vi "test1.vi"() -> ()   [LabVIEW 2017]
uses:
  <vilib>/userdefined/High Color/IMAQdx.ctl
  <vilib>/Platform/TimedLoop/XDataNode/timing_clust.ctl
  <vilib>/Platform/TimedLoop/XDataNode/nitl_modes.ctl
  <vilib>/Platform/TimedLoop/XDataNode/wakeup.ctl
  <vilib>/myRIO/Common/Instrument Driver Framework/myRIO v1.0/UART/vis/myRIO v1.0 Close UART.vi
  Global 1.vi
  Outputs.vi
  Inputs.vi
  <vilib>/myRIO/Common/Instrument Driver Framework/Utilities/vis/FPGA Ref Manager.vi
  <vilib>/myRIO/Common/Instrument Driver Framework/myRIO v1.0/myRIO v1.0 Reset FPGA.vi
  <vilib>/myRIO/Common/Instrument Driver Framework/myRIO v1.0/IRQ/vis/myRIO v1.0 IRQ Info FGV.vi
  <vilib>/myRIO/Common/Instrument Driver Framework/myRIO v1.0/IRQ/vis/myRIO v1.0 Timer IRQ Info FGV.vi
  <vilib>/myRIO/Common/Instrument Driver Framework/myRIO v1.0/IRQ/vis/myRIO v1.0 ISR Agent.vi
  <vilib>/platform/TimedLoop/XDataNode/XDataNode.xnode
  <vilib>/vision/driver/NI_Vision_Acquisition_Software.lvlib
  <vilib>/Platform/TimedLoop/XDataNode/XDNodeRunTimeDep.lvlib
  <vilib>/myRIO/Instrument Drivers/Utilities/Utilities.lvlib
panel:
  out "error out":errorcluster
  in  "Stop":bool
  out "Step":i16
  in  "Start":bool
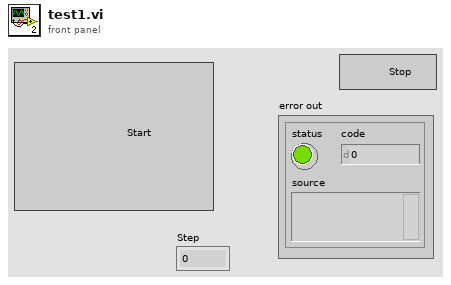
[diagram p1: front panel]
types:
  T1 = typedef "IMAQdx.ctl" = refnum<k21>
  T2 = typedef "XDNodeRunTimeDep.lvlib/timing_clust.ctl" = cluster{"Expected End [f-1]":u64, "Actual End [f-1]":u64, "Finished Late? [f-1]":bool, "Expected End [i-1]":u64, "Actual End [i-1]":u64, "Finished Late? [i-1]":bool, "Expected Start [i]":u64, "Actual Start [i]":u64, "Expected Start [f]":u64, "Actual Start [f]":u64, "Source Name":string, "Structure Name":string, "Period":i64, "Deadline":i64, "Offset":i64, "Start":i64, "Priority":i32, "Timeout":i32, "Mode":T3, "Wakeup Reason":T4, "Error":errorcluster, "Source Type":string, "Secondary Source Type":string, "Global End Time":u64, "Global Start Time":u64, "Frame Duration":u64, "Iteration Duration":u64, "Assigned CPU":i32, "I/O Scan Engine Mode":u32}
  T3 = typedef "XDNodeRunTimeDep.lvlib/nitl_modes.ctl" = enum32{"No Change", "Process missed periods, maintain original phase", "Discard missed periods, maintain original phase", "Process missed periods, ignore original phase", "Discard missed periods, ignore original phase"}
  T4 = typedef "XDNodeRunTimeDep.lvlib/wakeup.ctl" = enum32{"Normal", "Aborted", "Asynchronous wakeup", "Timing source error", "Timed loop error", "Timeout"}
  T5 = typedef "I2C.lvlib/I2C Reference.ctl" = cluster{"myRIO Reference":T6, "I2C Channels Enum":T10, "I2C Configuration":T11}
  T6 = typedef "myRIO Generic Hardware Reference.ctl" = cluster{"myRIO Model":T7, "myRIO Hardware Reference":T8}
  T7 = typedef "Hardware Version Enum.ctl" = enum16{"Unknown", "myRIO-1900", "myRIO-1950", "roboRIO", "NI ELVIS RIO CM"}
  T8 = typedef "myRIO v1.0 Reference.ctl" = cluster{"Generic FPGA Reference":T9, "Allow multiple opens":bool}
  T9 = typedef "Generic FPGA Reference.ctl" = refnum<k20>
  T10 = typedef "I2C Channels Enum.ctl" = enum16{"Not Connected", "A/I2C", "B/I2C", "I2C/I2C"}
  T11 = typedef "I2C.lvlib/I2C Configuration.ctl" = cluster{"I2C Transfer Rate":T12}
  T12 = typedef "I2C.lvlib/I2C Transfer Rate.ctl" = enum16{"Standard mode (100 kbps)", "Fast mode (400 kbps)"}
  T13 = typedef "IMAQ Image.ctl" = refnum<image>
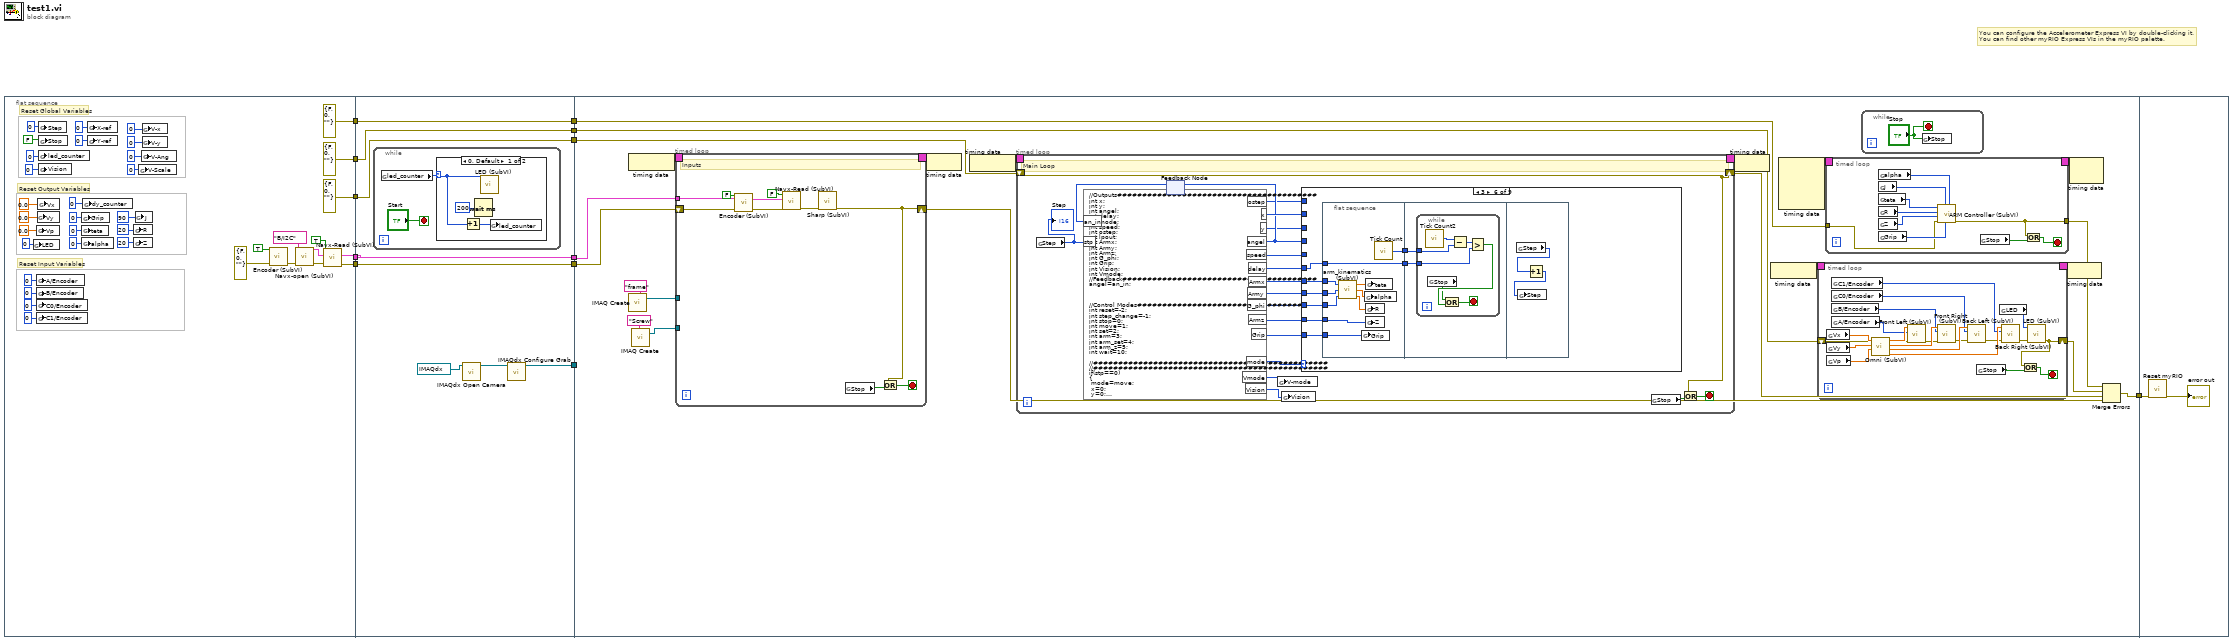
[diagram p0: block diagram]
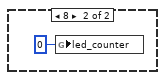
[diagram p2: hidden frame]
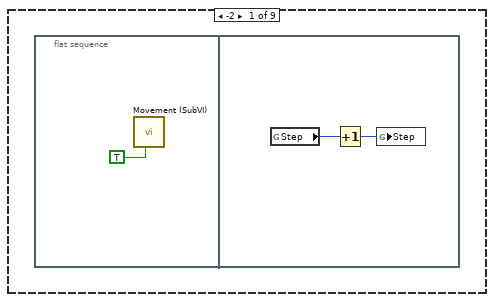
[diagram p3: hidden frame]
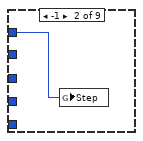
[diagram p4: hidden frame]
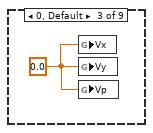
[diagram p5: hidden frame]
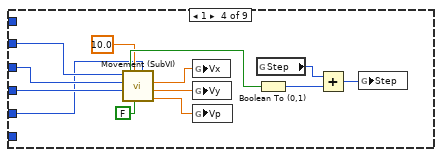
[diagram p6: hidden frame]
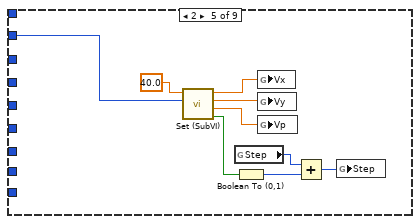
[diagram p7: hidden frame]
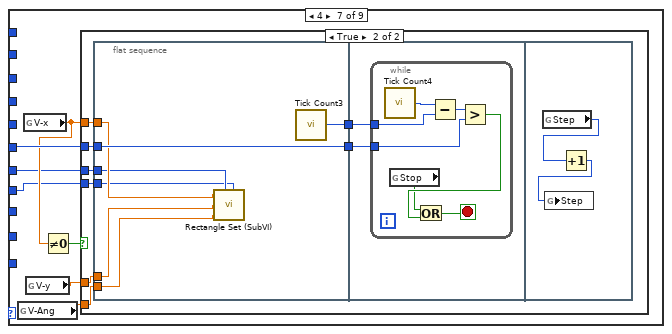
[diagram p8: hidden frame]
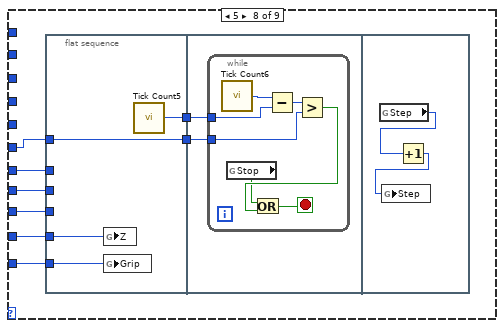
[diagram p10: hidden frame]
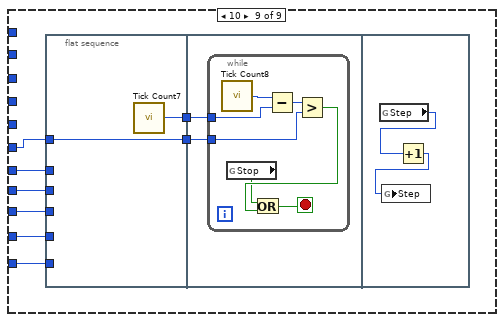
[diagram p11: hidden frame]
diagram:
  # "You can configure the Accelerometer Express VI by double-clicking it.\nYou can find other myRIO Express VIs in the myRIO palette."
  n1 = flat-sequence {
    tunnel: [w44] -> w12
    tunnel: [errorcluster {"status"=FALSE, "code"=0, "source"=""} ("error in (no error)")] -> w11
    tunnel: [errorcluster {"status"=FALSE, "code"=0, "source"=""} ("error in (no error)")] -> w10
    tunnel: [w42] -> w9
    tunnel: [errorcluster {"status"=FALSE, "code"=0, "source"=""} ("error in (no error)")] -> w8
    tunnel: w12 -> [w56]
    tunnel: [w56] -> w7
    tunnel: w11 -> [w55]
    tunnel: [w55] -> w6
    tunnel: w10 -> [w52]
    tunnel: w9 -> [w54]
    tunnel: [w54] -> w5
    tunnel: [w53] -> w4
    tunnel: w8 -> [w53]
    tunnel: [w52] -> w3
    tunnel: [w49] -> w2
    tunnel: w7 -> [w84]
    tunnel: w6 -> [w67]
    tunnel: w5 -> [w77]
    tunnel: w4 -> [w76]
    tunnel: [w75] -> w1
    tunnel: w3 -> [w68]
    tunnel: w2 -> [_]
    tunnel: w1 -> [w293]
    frame #0 {
      # "Reset Global Variables"
      # "Reset Input Variables"
      # "Reset Output Variables"
      # "Initialize"
      n2 = global write "Outputs.vi" "LED"(i8 0 ("LED")) -> ()
      n3 = global write "Outputs.vi" "Vp"(0.0 ("Vp")) -> ()
      n4 = global write "Inputs.vi" "A/Encoder"(0 ("A/Encoder")) -> ()
      n5 = global write "Inputs.vi" "B/Encoder"(0 ("B/Encoder")) -> ()
      n6 = global write "Inputs.vi" "C0/Encoder"(0 ("C0/Encoder")) -> ()
      n7 = global write "Inputs.vi" "C1/Encoder"(0 ("C1/Encoder")) -> ()
      n8 = global write "Outputs.vi" "Vy"(0.0 ("Vy")) -> ()
      n9 = global write "Outputs.vi" "Vx"(0.0 ("Vx")) -> ()
      n10 = global write "Global 1.vi" "Step"(i16 0 ("Step")) -> ()
      n11 = global write "Global 1.vi" "led_counter"(i8 0 ("Step")) -> ()
      n12 = global write "Global 1.vi" "Vision"(i8 0 ("Step")) -> ()
      n13 = global write "Global 1.vi" "Stop"(FALSE ("Stop")) -> ()
      n14 = global write "Outputs.vi" "Grip"(i16 0 ("Grip")) -> ()
      n15 = global write "Outputs.vi" "teta"(i16 0 ("teta")) -> ()
      n16 = global write "Outputs.vi" "alpha"(i16 0 ("alpha")) -> ()
      n17 = global write "Outputs.vi" "dy_counter"(i8 0 ("LED")) -> ()
      n18 = global write "Global 1.vi" "X-ref"(i64 0 ("X-ref")) -> ()
      n19 = global write "Global 1.vi" "Y-ref"(i64 0 ("Y-ref")) -> ()
      n20 = global write "Outputs.vi" "R"(i16 20 ("R")) -> ()
      n21 = global write "Outputs.vi" "Z"(i16 20 ("Z")) -> ()
      n22 = global write "Outputs.vi" "J"(i16 90 ("J")) -> ()
      n23 = global write "Global 1.vi" "V-Scale"(i64 0 ("Y-ref")) -> ()
      n24 = global write "Global 1.vi" "V-Ang"(i64 0 ("X-ref")) -> ()
      n25 = global write "Global 1.vi" "V-x"(i64 0 ("X-ref")) -> ()
      n26 = global write "Global 1.vi" "V-y"(i64 0 ("Y-ref")) -> ()
      n27 = call "Encoder (SubVI).vi"("error in (no error)"=errorcluster {"status"=FALSE, "code"=0, "source"=""}, "Reset?"=TRUE ("Reset Counter")) -> ("error out"=w26:errorcluster)  [unwired: 9 in]
      n28 = call "Navx-open (SubVI).vi"("error in (no error)"=w26, "Channel Name"=tag "B/I2C") -> ("error out"=w46:errorcluster, "I2C Ref Out"=w42:T5)  [unwired: 8 in]
      n29 = call "Navx-Read (SubVI).vi"("error in (no error)"=w46, "I2C Ref Out"=w42, "Reset"=TRUE) -> ("error out"=w44:errorcluster)  [unwired: 7 in, 1 out]
    }
    frame #1 {
      n30 = while {
        stop <- "Start" stop-if-true
        n31 = global read "Global 1.vi" "led_counter"() -> (w57:i8)
        n32 = case shown="0, Default" w57 {
          selector: w57 -> [w59 _]
          frame 0, Default {
            n33 = Increment(x=w59) -> (x+1=w61:i8)
            n34 = Wait (ms)(milliseconds to wait=u32 200) -> ()  [unwired: 1 out]
            n35 = call "LED (SubVI).vi"("LED"=w59) -> ()  [unwired: 10 in, 1 out]
            n36 = global write "Global 1.vi" "led_counter"(w61) -> ()
          }
          frame 8 {
            n37 = global write "Global 1.vi" "led_counter"(i8 0 ("led_counter")) -> ()
          }
        }
      }
      n38 = call <vilib>:"IMAQdx Open Camera.vi"("Session In"=T1 "cam0") -> ("Session Out"=w50:T1)  [unwired: 9 in, 1 out]
      n39 = call <vilib>:"IMAQdx Configure Grab.vi"("Session In"=w50) -> ("Session Out"=w49:T1)  [unwired: 9 in, 1 out]
    }
    frame #2 {
      n40 = call "IMAQ Create"("Image Name"="frame") -> ("New Image"=w64:T13)  [unwired: 4 in, 1 out]
      n41 = node-c288() -> (w79:T2)
      n42 = call "IMAQ Create"("Image Name"="Screw") -> ("New Image"=w63:T13)  [unwired: 4 in, 1 out]
      n43 = timed-loop {
        shift-right: [w103] -> w74
        shift-left: w84 -> [w107]
        timing: w79 -> [_]
        timing-out: [_] -> w78
        tunnel: w77 -> [w105]
        tunnel: w64 -> [_]
        tunnel: w63 -> [_]
        stop <- w106 stop-if-true
        # "Inputs"
        n44 = call "Encoder (SubVI).vi"("error in (no error)"=w107, "Reset?"=FALSE ("Boolean")) -> ("error out"=w101:errorcluster)  [unwired: 9 in]
        n45 = call "Navx-Read (SubVI).vi"("error in (no error)"=w101, "I2C Ref Out"=w105, "Reset"=FALSE) -> ("error out"=w100:errorcluster)  [unwired: 7 in, 1 out]
        n46 = call "Sharp (SubVI).vi"("error in (no error)"=w100) -> ("error out"=w103:errorcluster)  [unwired: 10 in]
        n47 = global read "Global 1.vi" "Stop"() -> (w104:bool)
        n48 = Or(x=w103, y=w104) -> (x .or. y?=w106:bool)
      }
      n49 = node-c288(w78) -> ()
      n50 = node-c288() -> (w81:T2)
      n51 = timed-loop {
        shift-right: [w129] -> w73
        shift-left: w68 -> [w129]
        timing: w81 -> [_]
        timing-out: [_] -> w80
        stop <- w130 stop-if-true
        # "Main Loop"
        n52 = global read "Global 1.vi" "Step"() -> (w122:i16)
        "Step" <- w122
        n53 = feedback #1() -> (w126:i32)  [unwired: 1 in]
        n54 = formula code="//Outputs########################################\nint x;\nint y;\nint angel;\nint delay;\nint mode;\nint speed;\nint ostep;\nint lpout;\nint Armx;\nint Army;\nint Armz;\nint G_phi;\nint Grip;\nint Vision;\nint Vmode;\n//Feedback#######################################\nangel=an_in;\n\n\n\n//Control Modes##################################\nint reset=-2;\nint step_change=-1; \nint stop=0;\nint move=1;\nint set=2;\nint arm=3;\nint arm_set=4;\nint arm_z=5;\nint wait=10;\n\n//###############################################\n//###############################################\nif(stp==0)\n{\n\tmode=move;\n\tx=0;\n\ty=0;\n\tangel=0;\n\tspeed=50;\n}\nif(stp==1)\n{\n\tmode=arm;\n\tArmx=75;\n\tArmy=0;\n\tArmz=180;\n\tdelay=4000;\n}\nif(stp==2)\n{\n\tmode=move;\n\tx=1000;\n\ty=0;\n\tangel=0;\n\tspeed=80;\n}\nif(stp==3)\n{\n\tmode=move;\n\tx=0;\n\ty=0;\n\tangel=-90;\n\tspeed=80;\n}\nif(stp==4)\n{\n\tmode=move;\n\tx=800;\n\ty=0;\n\tangel=0;\n\tspeed=80;\n}\nif(stp==5)\n{\n\tmode=set;\n\tx=3;\n\tspeed=50;\n}\nif(stp==6)\n{\n\tmode=reset;\n}\n\nif(stp==7)\n{\n\tmode=arm;\n\tArmx=75;\n\tArmy=0;\n\tArmz=280;\n\tdelay=4000;\n}\nif(stp==8)\n{\n\tVision=1;\n\tVmode=2;\n\tmode=wait;\n\tdelay=1000;\n}\nif(stp==9)\n{\n\tVision=1;\n\tVmode=2;\n\tmode=arm_set;\n\tArmx=75;\n\tArmy=0;\n\tdelay=4000;\n}\nif(stp==10)\n{\n\tVision=0;\n\tmode=wait;\n\tdelay=1000;\n}\nif(stp==11)\n{\n\tVision=0;\n\tmode=arm_z;\n\tArmz=100;\n\tGrip=0;\n\tdelay=3000;\n}\nif(stp==12)\n{\n\tmode=arm_z;\n\tArmz=100;\n\tGrip=1;\n\tdelay=1000;\n}\nif(stp==13)\n{\n\tmode=arm_z;\n\tArmz=200;\n\tGrip=1;\n\tdelay=1000;\n}\nif(stp==14)\n{\n\tmode=arm;\n\tArmx=75;\n\tArmy=0;\n\tArmz=200;\n\tGrip=1;\n\tdelay=4000;\n}\nif(stp==15)\n{\n\tmode=move;\n\tx=-1100;\n\ty=0;\n\tangel=0;\n\tspeed=80;\n}\nif(stp==16)\n{\n\tmode=move;\n\tx=0;\n\ty=0;\n\tangel=90;\n\tspeed=80;\n}\nif(stp==17)\n{\n\tmode=move;\n\tx=1250;\n\ty=0;\n\tangel=0;\n\tspeed=80;\n}\nif(stp==18)\n{\n\tmode=set;\n\tx=3;\n\tspeed=50;\n}\nif(stp==19)\n{\n\tmode=reset;\n}\nif(stp==20)\n{\n\tmode=arm_z;\n\tArmz=120;\n\tGrip=1;\n\tdelay=2000;\n}\nif(stp==21)\n{\n\tmode=arm_z;\n\tArmz=200;\n\tGrip=0;\n\tdelay=1000;\n}\n\n\nif(stp==22)\n{\n\tmode=stop;\n}"("stp"=w122, "an_in"=w126) -> ("x"=w128:i32, "y"=w123:i32, "mode"=w119:i32, "angel"=w125:i32, "delay"=w127:i32, "speed"=w124:i32, "ostep"=w120:i32, "Armx"=w117:i32, "Army"=w116:i32, "Armz"=w115:i32, "G_phi"=w118:i32, "Grip"=w114:i32, "Vision"=w113:i32, "Vmode"=w112:i32)
        n55 = feedback-in #1(w125) -> ()
        n56 = global write "Global 1.vi" "V-mode"(w112) -> ()
        n57 = global write "Global 1.vi" "Vision"(w113) -> ()
        n58 = case shown="3" w119 {
          tunnel: w128 -> [_ _ _ w142 w157 _ _ _ _]
          tunnel: w123 -> [_ _ _ w141 _ _ _ _ _]
          tunnel: w125 -> [_ _ _ w140 _ _ _ _ _]
          tunnel: w127 -> [_ _ _ _ _ w164 w193 w226 w249]
          tunnel: w124 -> [_ _ _ w139 _ _ _ _ _]
          tunnel: w120 -> [_ w134 _ _ _ _ _ _ _]
          tunnel: w118 -> [_ _ _ _ _ w160 _ w222 w245]
          tunnel: w117 -> [_ _ _ _ _ w162 w188 w224 w247]
          tunnel: w116 -> [_ _ _ _ _ w161 w187 w223 w246]
          tunnel: w115 -> [_ _ _ _ _ w159 _ w221 w244]
          tunnel: w114 -> [_ _ _ _ _ w158 _ w220 w243]
          frame -2 {
            n59 = flat-sequence {
              frame #0 {
                n60 = call "Movement (SubVI).vi"("Reset"=TRUE) -> ()  [unwired: 6 in, 4 out]
              }
              frame #1 {
                n61 = global read "Global 1.vi" "Step"() -> (w133:i16)
                n62 = Increment(x=w133) -> (x+1=w132:i16)
                n63 = global write "Global 1.vi" "Step"(w132) -> ()
              }
            }
          }
          frame -1 {
            n64 = global write "Global 1.vi" "Step"(w134) -> ()
          }
          frame 0, Default {
            w135 = 0.0 ("Vy")
            n65 = global write "Outputs.vi" "Vx"(w135) -> ()
            n66 = global write "Outputs.vi" "Vy"(w135) -> ()
            n67 = global write "Outputs.vi" "Vp"(w135) -> ()
          }
          frame 1 {
            n68 = call "Movement (SubVI).vi"("Speed"=w139, "Reset"=FALSE, "Acc"=10.0, "Goal P"=w140, "Goal Y"=w141, "Goal X"=w142) -> ("Vp"=w144:dbl, "Vy"=w145:dbl, "Vx"=w146:dbl, "Reach?"=w147:bool)  [unwired: 1 in]
            n69 = global write "Outputs.vi" "Vx"(w146) -> ()
            n70 = global write "Outputs.vi" "Vy"(w145) -> ()
            n71 = global write "Outputs.vi" "Vp"(w144) -> ()
            n72 = global read "Global 1.vi" "Step"() -> (w136:i16)
            n73 = Boolean To (0,1)(Boolean=w147) -> (0, 1=w148:i16)
            n74 = Add(x=w136, y=w148) -> (x+y=w137:i16)
            n75 = global write "Global 1.vi" "Step"(w137) -> ()
          }
          frame 2 {
            n76 = call "Set (SubVI).vi"("Mode"=w157, "speed"=40.0) -> ("Reach?"=w149:bool, "Vp"=w153:dbl, "Vy"=w154:dbl, "Vx"=w155:dbl)  [unwired: 4 in]
            n77 = global read "Global 1.vi" "Step"() -> (w150:i16)
            n78 = Boolean To (0,1)(Boolean=w149) -> (0, 1=w152:i16)
            n79 = global write "Outputs.vi" "Vx"(w155) -> ()
            n80 = global write "Outputs.vi" "Vy"(w154) -> ()
            n81 = global write "Outputs.vi" "Vp"(w153) -> ()
            n82 = Add(x=w150, y=w152) -> (x+y=w151:i16)
            n83 = global write "Global 1.vi" "Step"(w151) -> ()
          }
          frame 3 {
            n84 = flat-sequence {
              tunnel: [w175] -> w165
              tunnel: w164 -> [w171]
              tunnel: [w171] -> w163
              tunnel: w162 -> [w170]
              tunnel: w161 -> [w169]
              tunnel: w160 -> [w168]
              tunnel: w159 -> [w167]
              tunnel: w158 -> [w166]
              tunnel: w165 -> [w177]
              tunnel: w163 -> [w176]
              frame #0 {
                n85 = call "arm_kinematics (SubVI).vi"("alpha"=w168, "y"=w169, "x"=w170) -> ("R"=w172:dbl, "alpha"=w173:dbl, "teta"=w174:dbl)
                n86 = global write "Outputs.vi" "Grip"(w166) -> ()
                n87 = global write "Outputs.vi" "alpha"(w173) -> ()
                n88 = global write "Outputs.vi" "teta"(w174) -> ()
                n89 = global write "Outputs.vi" "R"(w172) -> ()
                n90 = global write "Outputs.vi" "Z"(w167) -> ()
                n91 = call "Tick Count"() -> ("Tick Count(mSec)"=w175:u32)
              }
              frame #1 {
                n92 = while {
                  tunnel: w177 -> [w183]
                  tunnel: w176 -> [w178]
                  stop <- w180 stop-if-true
                  n93 = call "Tick Count2"() -> ("Tick Count(mSec)"=w184:u32)
                  n94 = global read "Global 1.vi" "Stop"() -> (w179:bool)
                  n95 = Subtract(x=w184, y=w183) -> (x-y=w182:u32)
                  n96 = Greater?(x=w182, y=w178) -> (0:w181:bool)
                  n97 = Or(x=w179, y=w181) -> (x .or. y?=w180:bool)
                }
              }
              frame #2 {
                n98 = global read "Global 1.vi" "Step"() -> (w185:i16)
                n99 = Increment(x=w185) -> (x+1=w186:i16)
                n100 = global write "Global 1.vi" "Step"(w186) -> ()
              }
            }
          }
          frame 4 {
            n101 = global read "Global 1.vi" "V-Ang"() -> (w189:sgl)
            n102 = global read "Global 1.vi" "V-x"() -> (w190:sgl)
            n103 = global read "Global 1.vi" "V-y"() -> (w192:sgl)
            n104 = Not Equal To 0?(x=w190) -> (x != 0?=w191:bool)
            n105 = case shown="True" w191 {
              tunnel: w193 -> [_ w199]
              tunnel: w192 -> [_ w198]
              tunnel: w190 -> [_ w197]
              tunnel: w189 -> [_ w196]
              tunnel: w188 -> [_ w195]
              tunnel: w187 -> [_ w194]
              frame False {
              }
              frame True {
                n106 = flat-sequence {
                  tunnel: [w208] -> w201
                  tunnel: w199 -> [w207]
                  tunnel: [w207] -> w200
                  tunnel: w198 -> [w205]
                  tunnel: w197 -> [w206]
                  tunnel: w196 -> [w204]
                  tunnel: w195 -> [w203]
                  tunnel: w194 -> [w202]
                  tunnel: w201 -> [w210]
                  tunnel: w200 -> [w209]
                  frame #0 {
                    n107 = call "Rectangle Set (SubVI).vi"("x"=w206, "x in"=w203, "y"=w205, "alpha"=w204, "y in"=w202) -> ()  [unwired: 6 in]
                    n108 = call "Tick Count3"() -> ("Tick Count(mSec)"=w208:u32)
                  }
                  frame #1 {
                    n109 = while {
                      tunnel: w210 -> [w216]
                      tunnel: w209 -> [w211]
                      stop <- w213 stop-if-true
                      n110 = call "Tick Count4"() -> ("Tick Count(mSec)"=w217:u32)
                      n111 = global read "Global 1.vi" "Stop"() -> (w212:bool)
                      n112 = Subtract(x=w217, y=w216) -> (x-y=w215:u32)
                      n113 = Greater?(x=w215, y=w211) -> (0:w214:bool)
                      n114 = Or(x=w212, y=w214) -> (x .or. y?=w213:bool)
                    }
                  }
                  frame #2 {
                    n115 = global read "Global 1.vi" "Step"() -> (w218:i16)
                    n116 = Increment(x=w218) -> (x+1=w219:i16)
                    n117 = global write "Global 1.vi" "Step"(w219) -> ()
                  }
                }
              }
            }
          }
          frame 5 {
            n118 = flat-sequence {
              tunnel: [w231] -> w227
              tunnel: w226 -> [w230]
              tunnel: [w230] -> w225
              tunnel: w224 -> [_]
              tunnel: w223 -> [_]
              tunnel: w222 -> [_]
              tunnel: w221 -> [w229]
              tunnel: w220 -> [w228]
              tunnel: w227 -> [w233]
              tunnel: w225 -> [w232]
              frame #0 {
                n119 = global write "Outputs.vi" "Z"(w229) -> ()
                n120 = global write "Outputs.vi" "Grip"(w228) -> ()
                n121 = call "Tick Count5"() -> ("Tick Count(mSec)"=w231:u32)
              }
              frame #1 {
                n122 = while {
                  tunnel: w233 -> [w239]
                  tunnel: w232 -> [w234]
                  stop <- w236 stop-if-true
                  n123 = call "Tick Count6"() -> ("Tick Count(mSec)"=w240:u32)
                  n124 = global read "Global 1.vi" "Stop"() -> (w235:bool)
                  n125 = Subtract(x=w240, y=w239) -> (x-y=w238:u32)
                  n126 = Greater?(x=w238, y=w234) -> (0:w237:bool)
                  n127 = Or(x=w235, y=w237) -> (x .or. y?=w236:bool)
                }
              }
              frame #2 {
                n128 = global read "Global 1.vi" "Step"() -> (w241:i16)
                n129 = Increment(x=w241) -> (x+1=w242:i16)
                n130 = global write "Global 1.vi" "Step"(w242) -> ()
              }
            }
          }
          frame 10 {
            n131 = flat-sequence {
              tunnel: [w252] -> w250
              tunnel: w249 -> [w251]
              tunnel: [w251] -> w248
              tunnel: w247 -> [_]
              tunnel: w246 -> [_]
              tunnel: w245 -> [_]
              tunnel: w244 -> [_]
              tunnel: w243 -> [_]
              tunnel: w250 -> [w254]
              tunnel: w248 -> [w253]
              frame #0 {
                n132 = call "Tick Count7"() -> ("Tick Count(mSec)"=w252:u32)
              }
              frame #1 {
                n133 = while {
                  tunnel: w254 -> [w260]
                  tunnel: w253 -> [w255]
                  stop <- w257 stop-if-true
                  n134 = call "Tick Count8"() -> ("Tick Count(mSec)"=w261:u32)
                  n135 = global read "Global 1.vi" "Stop"() -> (w256:bool)
                  n136 = Subtract(x=w261, y=w260) -> (x-y=w259:u32)
                  n137 = Greater?(x=w259, y=w255) -> (0:w258:bool)
                  n138 = Or(x=w256, y=w258) -> (x .or. y?=w257:bool)
                }
              }
              frame #2 {
                n139 = global read "Global 1.vi" "Step"() -> (w262:i16)
                n140 = Increment(x=w262) -> (x+1=w263:i16)
                n141 = global write "Global 1.vi" "Step"(w263) -> ()
              }
            }
          }
        }
        n142 = global read "Global 1.vi" "Stop"() -> (w121:bool)
        n143 = Or(x=w129, y=w121) -> (x .or. y?=w130:bool)
      }
      n144 = node-c288(w80) -> ()
      n145 = node-c288() -> (w83:T2)
      n146 = node-c288() -> (w71:T2)  [unwired: 4 in]
      n147 = timed-loop {
        timing: w83 -> [_]
        timing-out: [_] -> w82
        shift-right: [w269] -> w72
        shift-left: w76 -> [w276]
        stop <- w284 stop-if-true
        n148 = global read "Outputs.vi" "Vx"() -> (w283:dbl)
        n149 = global read "Outputs.vi" "Vy"() -> (w286:dbl)
        n150 = global read "Outputs.vi" "Vp"() -> (w285:dbl)
        n151 = global read "Inputs.vi" "C1/Encoder"() -> (w275:i32)
        n152 = global read "Inputs.vi" "C0/Encoder"() -> (w274:i32)
        n153 = global read "Inputs.vi" "B/Encoder"() -> (w273:i32)
        n154 = global read "Inputs.vi" "A/Encoder"() -> (w272:i32)
        n155 = call "Omni (SubVI).vi"("Vp"=w285, "Vy"=w286, "Vx"=w283) -> ("Back_Right"=w281:dbl, "Back_Left"=w287:dbl, "Front_Right"=w282:dbl, "Front_Left"=w279:dbl)  [unwired: 4 in]
        n156 = call "Front Left (SubVI).vi"("setpoint"=w279, "Counter Value"=w272, "error in"=w276) -> ("error out"=w280:errorcluster)  [unwired: 6 in, 1 out]
        n157 = call "Front Right (SubVI).vi"("error in"=w280, "Counter Value"=w273, "setpoint"=w282) -> ("error out"=w278:errorcluster)  [unwired: 7 in, 1 out]
        n158 = call "Back Left (SubVI).vi"("error in"=w278, "Counter Value"=w274, "setpoint"=w287) -> ("error out"=w277:errorcluster)  [unwired: 7 in, 1 out]
        n159 = global read "Global 1.vi" "Stop"() -> (w271:bool)
        n160 = global read "Outputs.vi" "LED"() -> (w268:i8)
        n161 = call "Back Right (SubVI).vi"("error in"=w277, "Counter Value"=w275, "setpoint"=w281) -> ("error out"=w270:errorcluster)  [unwired: 7 in, 1 out]
        n162 = call "LED (SubVI).vi"("error in (no error)"=w270, "LED"=w268) -> ("error out"=w269:errorcluster)  [unwired: 9 in]
        n163 = Or(x=w269, y=w271) -> (x .or. y?=w284:bool)
      }
      n164 = timed-loop {
        timing: w71 -> [_]
        timing-out: [_] -> w70
        tunnel: w67 -> [w88]
        tunnel: [w85] -> w69
        stop <- w86 stop-if-true
        n165 = global read "Outputs.vi" "alpha"() -> (w89:i16)
        n166 = global read "Outputs.vi" "J"() -> (w90:i16)
        n167 = global read "Outputs.vi" "teta"() -> (w94:i16)
        n168 = global read "Outputs.vi" "R"() -> (w93:i16)
        n169 = global read "Outputs.vi" "Z"() -> (w92:i16)
        n170 = global read "Outputs.vi" "Grip"() -> (w91:i16)
        n171 = call "ARM Controller (SubVI).vi"("alpha"=w89, "Grip"=w91, "J"=w90, "error in (no error)"=w88, "Z"=w92, "R"=w93, "teta"=w94) -> ("error out"=w85:errorcluster)  [unwired: 4 in]
        n172 = global read "Global 1.vi" "Stop"() -> (w87:bool)
        n173 = Or(x=w85, y=w87) -> (x .or. y?=w86:bool)
      }
      n174 = while {
        stop <- "Stop" stop-if-true
        n175 = global write "Global 1.vi" "Stop"("Stop") -> ()
      }
      n176 = node-c288(w82) -> ()
      n177 = node-c288(w70) -> ()  [unwired: 1 out]
      n178 = Merge Errors(w69, w72, w73, w74) -> (w75:errorcluster)
    }
    frame #3 {
      # "Close"
      n179 = call <vilib>:"Reset myRIO.vi"("error in (no error)"=w293) -> ("error out"=→"error out":errorcluster)  [unwired: 10 in]
    }
  }
